vi "Exit While Loop.vi"(0 "Diagram in":refnum<vi>, 1 "Conditional Terminals":refnum<vi>[](array[refnum]), 2 "Loop Terminal Types":T1[](array[typedef]), 5 "Outputs":refnum<vi>[](array[refnum]), 7 "Shift Registers":refnum<vi>[](array[refnum]), 9 "Stop Condition":refnum<vi>, 11 "error in (no error)":errorcluster) -> (4 "Diagram out":refnum<vi>, 6 "Outputs":refnum<vi>[](array[refnum]), 8 "Shift Registers":refnum<vi>[](array[refnum]), 15 "error out":errorcluster)   [LabVIEW 2015, in "Scripting.lvlib"]
doc: "Exits the While Loop that owns <B>Diagram in</B>, supplying the structure's owning diagram at <B>Diagram out</B>.\n\n<B>Stop Condition</B> is the terminal to wire to the conditional terminal of the While Loop.\n\n<B>Conditional Terminals</B> is optionally an array of terminals to wire to the conditional terminal of the While Loop's output tunnels.\n\n<B>Loop Terminal Types</B> is optionally and array of terminal types of the While Loop's output tunnels."
uses:
  Scripting.lvlib
  Loop Terminal Type.ctl
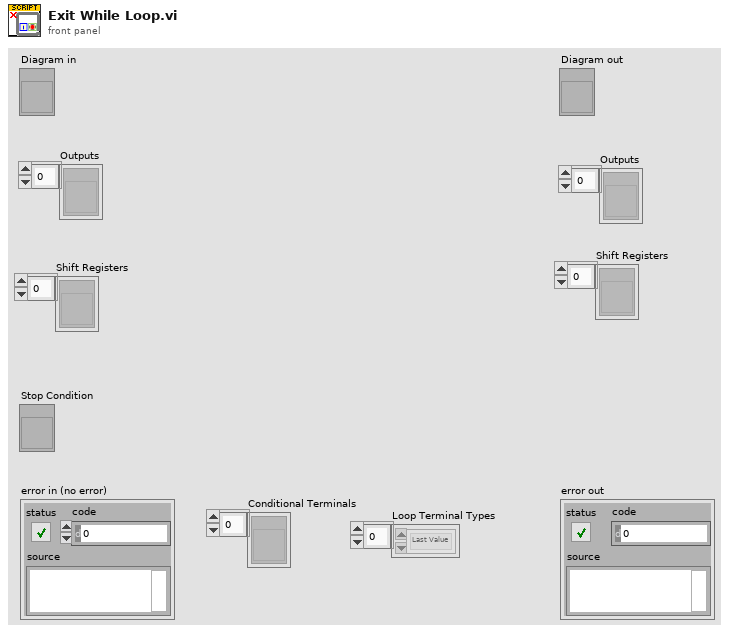
[diagram p1: front panel]
types:
  T1 = typedef "Scripting.lvlib/Loop Terminal Type.ctl" = enum16{"Last Value", "Indexing", "Concatenating"}
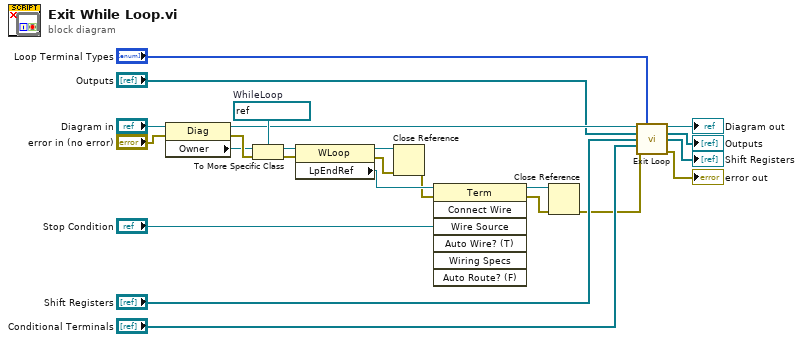
[diagram p0: block diagram]
diagram:
  w23 = refnum<vi> refnum  # WhileLoop
  n1 = property class="Diag"(reference="Diagram in", error in="error in (no error)") -> (reference out=w19:refnum<vi>, error out=w24:errorcluster, "Owner"=w22:refnum<vi>)
  n2 = To More Specific Class(target class=w23, reference=w22, error in=w24) -> (specific class reference=w13:refnum<vi>, error out=w12:errorcluster)
  n3 = property class="WLoop"(reference=w13, error in=w12) -> (reference out=w3:refnum<vi>, error out=w6:errorcluster, "LpEndRef"=w7:refnum<vi>)
  n4 = Close Reference(reference=w3, error in (no error)=w6) -> (error out=w4:errorcluster)
  n5 = invoke class="Term" method="Connect Wire"(reference=w7, error in=w4, "Wire Source"="Stop Condition") -> (reference out=w1:refnum<vi>, error out=w9:errorcluster)  [unwired: 4 in, 5 out]
  n6 = Close Reference(reference=w1, error in (no error)=w9) -> (error out=w2:errorcluster)
  n7 = call "Exit Loop.vi"("Diagram in"=w19, "Loop Terminal Types"="Loop Terminal Types", "Outputs"="Outputs", "Shift Registers"="Shift Registers", "Conditional Terminals"="Conditional Terminals", "error in (no error)"=w2) -> ("Diagram out"=→"Diagram out":refnum<vi>, "Outputs"=→"Outputs":refnum<vi>[], "Shift Registers"=→"Shift Registers":refnum<vi>[], "error out"=→"error out":errorcluster)  [unwired: 6 in]
